vi "pockels_power_estimate.vi"(8 "error in":errorcluster, 10 "Pockels calibration":T1, 11 "Pockels volt":dbl) -> (0 "error out":errorcluster, 3 "Power estimate":dbl)   [LabVIEW 2011, in "Fiberscope_library.lvlib"]
uses:
  Fiberscope_library.lvlib
  typedefs/pockels_calibration_cluster.ctl
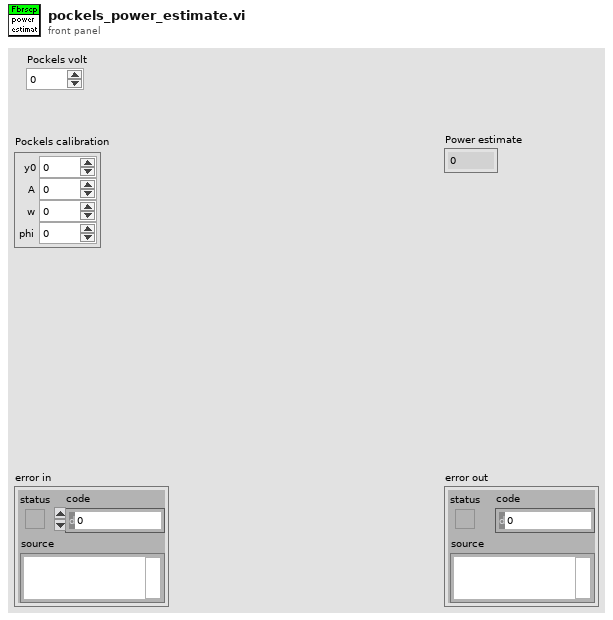
[diagram p1: front panel]
types:
  T1 = typedef "Fiberscope_library.lvlib/pockels_calibration_cluster.ctl" = cluster{"y0":dbl, "A":dbl, "w":dbl, "phi":dbl}
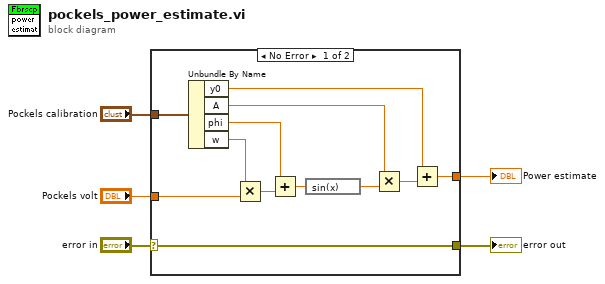
[diagram p0: block diagram]
diagram:
  n1 = case shown="No Error" "error in" {
    selector: "error in" -> [w17 w18]
    tunnel: [w17 w18] -> w4
    tunnel: "Pockels volt" -> [w14 _]
    tunnel: "Pockels calibration" -> [w16 _]
    tunnel: [w6 _] -> w1
    frame No Error {
      n2 = Unbundle By Name(w16) -> ("y0"=w7:dbl, "A"=w9:dbl, "phi"=w12:dbl, "w"=w15:dbl)
      n3 = Multiply(x=w15, y=w14) -> (x*y=w13:dbl)
      n4 = Add(x=w12, y=w13) -> (x+y=w11:dbl)
      n5 = expression code="sin(x)"(w11) -> (w10:dbl)
      n6 = Multiply(x=w9, y=w10) -> (x*y=w8:dbl)
      n7 = Add(x=w7, y=w8) -> (x+y=w6:dbl)
    }
    frame Error {
    }
  }
  "error out" <- w4
  "Power estimate" <- w1
